vi "응답 Parsing.vi"(1 "응답 프레임":string="\u000600RSB0164100020003000400050006000700080009000A0000000000000000000000000000000000000000000000000000000000000000000000000000000000000000000000000000000000000000000000000000000000000000000000000000000000000000000\u0003") -> (0 "U16배열":u16[](array[numeric]))   [LabVIEW 2014]
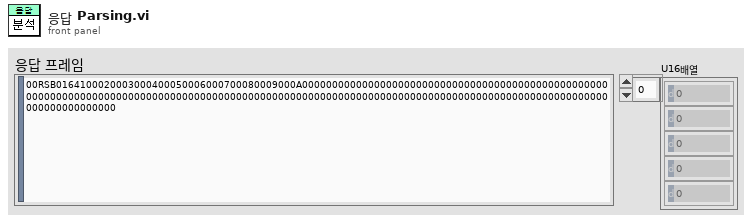
[diagram p1: front panel]
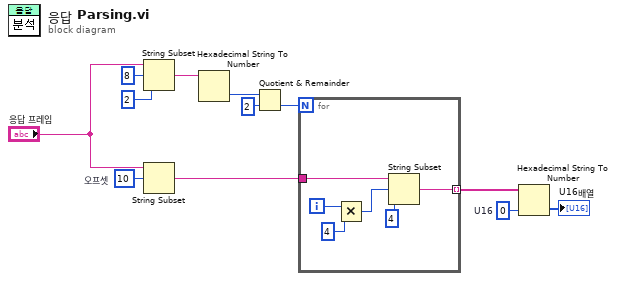
[diagram p0: block diagram]
diagram:
  w2 = u16 0  # U16
  w8 = 10  # 오프셋
  n1 = String Subset(string="응답 프레임", offset (0)=8 ("오프셋(0)"), length (rest)=2 ("길이(나머지)")) -> (substring=w10:string)
  n2 = String Subset(string="응답 프레임", offset (0)=w8) -> (substring=w4:string)  [unwired: 1 in]
  n3 = Hexadecimal String To Number(string=w10) -> (number=w7:u32)  [unwired: 2 in, 1 out]
  n4 = Quotient & Remainder(x=w7, y=u32 2) -> (floor(x/y)=w5:u32)  [unwired: 1 out]
  n5 = for {
    N: w5 -> [_]
    tunnel: w4 -> [w18]
    tunnel: [w13] -> w3 mode=indexing
    i -> [w17]
    n6 = Multiply(x=w17, y=4) -> (x*y=w15:i32)
    n7 = String Subset(string=w18, offset (0)=w15, length (rest)=4 ("길이(나머지)")) -> (substring=w13:string)
  }
  n8 = Hexadecimal String To Number(string=w3, default (0uL)=w2) -> (number=→"U16배열":u16[])  [unwired: 1 in, 1 out]
